vi "Open VI Block Diagram.vi"(8 "error in (no error)":errorcluster, 11 "VI in":refnum<vi>) -> (0 "error out":errorcluster, 3 "VI out":refnum<vi>)   [LabVIEW 2019, in "Panther Dashboard.lvlib"]
uses:
  Panther Dashboard.lvlib
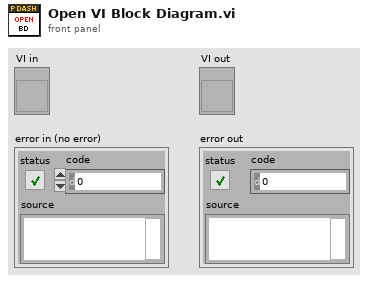
[diagram p1: front panel]
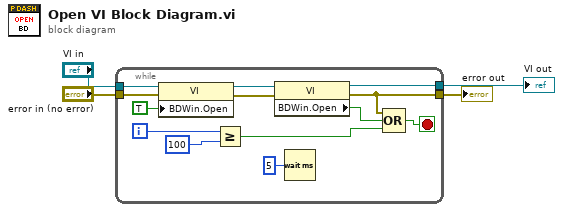
[diagram p0: block diagram]
diagram:
  n1 = while {
    tunnel: [w13] -> w4
    tunnel: [w15] -> w1
    tunnel: "VI in" -> [w12]
    tunnel: "error in (no error)" -> [w17]
    i -> [w9]
    stop <- w7 stop-if-true
    n2 = property class="VI"(reference=w12, error in=w17, "BDWin.Open"=TRUE ("Block Diagram Window:Open")) -> (reference out=w10:refnum<vi>, error out=w16:errorcluster)
    n3 = Greater Or Equal?(x=w9, y=100) -> (x >= y?=w6:bool)
    n4 = property class="VI"(reference=w10, error in=w16) -> (reference out=w13:refnum<vi>, error out=w15:errorcluster, "BDWin.Open"=w14:bool)
    n5 = Wait (ms)(milliseconds to wait=u32 5) -> ()  [unwired: 1 out]
    n6 = Compound Arithmetic op=OR(w15, w14, w6) -> (w7:bool)
  }
  "VI out" <- w4
  "error out" <- w1
